vi "Append Report Text.vi"   [LabVIEW 2015, in "NI_report.lvclass"]
doc: "Appends text to the selected report. Wire data to the <B>text</B> input to determine the polymorphic instance to use or manually select the instance."
uses:
  <vilib>/Utility/NIReport.llb/NI_report.lvclass
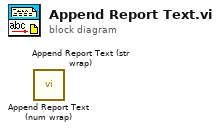
[diagram p0: block diagram]
diagram:
  n1 = call <vilib>:"Append Report Text (num wrap).vi"() -> ()  [unwired: 12 in, 4 out]
  n2 = call <vilib>:"Append Report Text (str wrap).vi"() -> ()  [unwired: 12 in, 4 out]
